vi "open MB.vi"(8 "error in (no error)":errorcluster caption="错误输入（无错误）", 10 "VISA Resource":refnum<visa-resource-name>, 11 "HL7 输入":refnum<class "HL7.lvclass">) -> (0 "error out":errorcluster caption="错误输出", 3 "HL7 输出":refnum<class "HL7.lvclass">)   [LabVIEW 2016, in "HL7.lvlib" / "HL7.lvclass"]
uses:
  HL7.lvclass
  <vilib>/Plasmionique/MB Master/MB_Master_Serial/MB_Master_Serial.lvclass
  C:/Program Files (x86)/National Instruments/LabVIEW 2016/vi.lib/Plasmionique/MB Master/MB_Master/MB_Master.lvclass
  <vilib>/Plasmionique/MB Master/MB_Master/MB_Master.lvclass
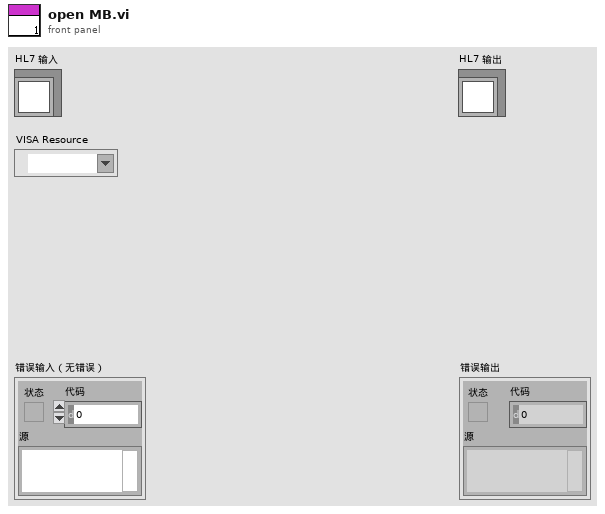
[diagram p1: front panel]
types:
  T1 = cluster{"baud rate (bps)":u32, "stop bits":u16, "parity":u16, "flow control":u16, "timeout":u32, "retries":i32}
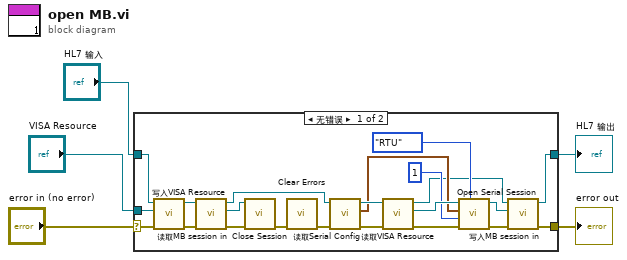
[diagram p0: block diagram]
diagram:
  n1 = case shown="无错误" "error in (no error)" {
    selector: "error in (no error)" -> [w10 w29]
    tunnel: [w11 w29] -> w4
    tunnel: [w12 w28] -> w2
    tunnel: "HL7 输入" -> [w7 w28]
    tunnel: "VISA Resource" -> [w6 _]
    frame No Error {
      n2 = call-dynamic "写入VISA Resource.vi"("error in (no error)"=w10, "VISA Resource"=w6, "HL7输入"=w7) -> ("error out"=w9:errorcluster, "HL7输出"=w8:refnum<class "HL7.lvclass">)  [unwired: 7 in]
      n3 = call-dynamic "读取MB session in.vi"("error in (no error)"=w9, "HL7输入"=w8) -> ("error out"=w26:errorcluster, "MB Serial Master:MB_Master"=w27:refnum<class "MB_Master.lvclass">, "HL7输出"=w24:refnum<class "HL7.lvclass">)  [unwired: 7 in]
      n4 = call-dynamic "Close Session.vi"("error in (no error)"=w26, "MB session in"=w27) -> ("error out"=w25:errorcluster)  [unwired: 9 in]
      n5 = call <vilib>:"Clear Errors.vi"("error in (no error)"=w25) -> ("error out"=w23:errorcluster)  [unwired: 5 in, 1 out]
      n6 = call-dynamic "读取Serial Config.vi"("error in (no error)"=w23, "HL7输入"=w24) -> ("error out"=w19:errorcluster, "Serial Config"=w20:T1, "HL7输出"=w22:refnum<class "HL7.lvclass">)  [unwired: 7 in]
      n7 = call-dynamic "读取VISA Resource.vi"("error in (no error)"=w19, "HL7输入"=w22) -> ("error out"=w18:errorcluster, "VISA Resource"=w21:refnum<visa-resource-name>, "HL7输出"=w13:refnum<class "HL7.lvclass">)  [unwired: 7 in]
      n8 = call <vilib>:"Open Serial Session.vi"("Mode (RTU)"=enum16{"RTU", "ASCII"}."RTU", "Error in"=w18, "Slave ID"=u8 1, "Serial Config"=w20, "VISA Resource"=w21) -> ("Error out"=w15:errorcluster, "MB_Serial session"=w14:refnum<class "MB_Master_Serial.lvclass">)  [unwired: 5 in]
      n9 = call-dynamic "写入MB session in.vi"("error in (no error)"=w15, "MB Serial Master:MB_Master"=w14, "HL7输入"=w13) -> ("error out"=w11:errorcluster, "HL7输出"=w12:refnum<class "HL7.lvclass">)  [unwired: 7 in]
    }
    frame Error {
    }
  }
  "error out" <- w4
  "HL7 输出" <- w2
